vi "Autosize Columns.vi"(0 "Active VI Info":T3, 5 "Options":T1={"Whitespace Border"=10, "Resize Table"=FALSE, "Number of Columns"=20, "Default Width"=50}, 7 "Menu Selection":T2, 11 "error in (no error)":errorcluster) -> (15 "error out":errorcluster)   [LabVIEW 2015]
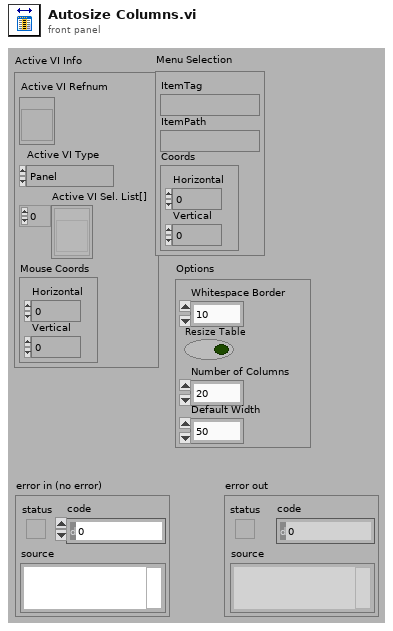
[diagram p1: front panel]
types:
  T1 = cluster{"Whitespace Border":i16, "Resize Table":bool, "Number of Columns":i32, "Default Width":u32}
  T2 = cluster{"ItemTag":string, "ItemPath":string, "Coords":cluster{"Horizontal":i32, "Vertical":i32}}
  T3 = cluster{"Active VI Refnum":refnum<vi>, "Active VI Type":enum16{"Panel", "Diagram"}, "Active VI Sel. List[]":refnum<vi>[], "Mouse Coords":cluster{"Horizontal":i32, "Vertical":i32}}
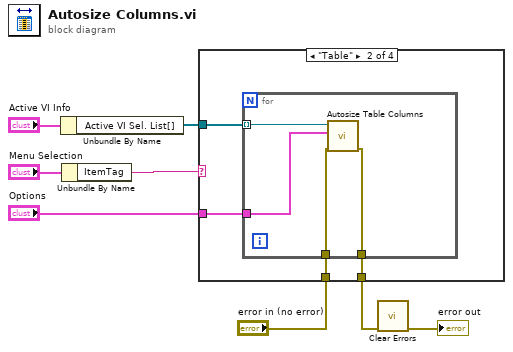
[diagram p0: block diagram]
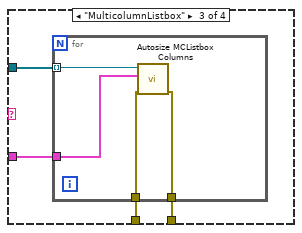
[diagram p3: hidden frame]
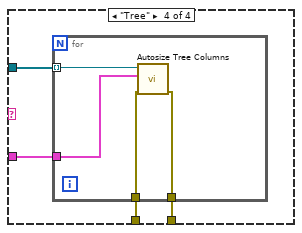
[diagram p4: hidden frame]
diagram:
  n1 = Unbundle By Name("Active VI Info") -> ("Active VI Sel. List[]"=w5:refnum<vi>[])
  n2 = Unbundle By Name("Menu Selection") -> ("ItemTag"=w7:string)
  n3 = case shown="\"Table\"" w7 {
    tunnel: w5 -> [_ w13 w21 w29]
    tunnel: "error in (no error)" -> [w9 w12 w20 w28]
    tunnel: [w9 w11 w19 w27] -> w3
    tunnel: "Options" -> [_ w10 w18 w26]
    frame Default {
    }
    frame "Table" {
      n4 = for {
        tunnel: w13 -> [w17] mode=indexing
        tunnel: w12 -> [w16]
        tunnel: [w15] -> w11
        tunnel: w10 -> [w14]
        n5 = call "Autosize Table Columns.vi"("error in (no error)"=w16, "Options"=w14, "Table Ref"=w17) -> ("error out"=w15:errorcluster)  [unwired: 1 in, 3 out]
      }
    }
    frame "MulticolumnListbox" {
      n6 = for {
        tunnel: w21 -> [w23] mode=indexing
        tunnel: w20 -> [w25]
        tunnel: [w24] -> w19
        tunnel: w18 -> [w22]
        n7 = call "Autosize MCListbox Columns.vi"("error in (no error)"=w25, "Options"=w22, "Multicolumn Ref"=w23) -> ("error out"=w24:errorcluster)  [unwired: 2 in, 2 out]
      }
    }
    frame "Tree" {
      n8 = for {
        tunnel: w29 -> [w31] mode=indexing
        tunnel: w28 -> [w33]
        tunnel: [w32] -> w27
        tunnel: w26 -> [w30]
        n9 = call "Autosize Tree Columns.vi"("error in (no error)"=w33, "Options"=w30, "Tree Ref"=w31) -> ("error out"=w32:errorcluster)  [unwired: 4 out]
      }
    }
  }
  n10 = call <vilib>:"Clear Errors.vi"("error in (no error)"=w3) -> ("error out"=→"error out":errorcluster)  [unwired: 1 in, 5 out]
